vi "deadbands and cubic drive.vi"(8 "Axis2":dbl, 11 "Axis1":dbl) -> (0 "Axis2":dbl, 3 "Axis1":dbl)   [LabVIEW 2017]
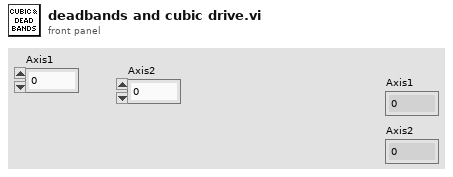
[diagram p1: front panel]
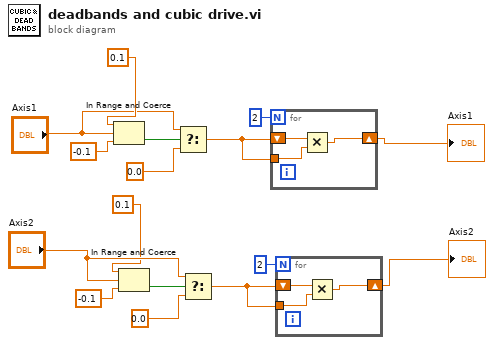
[diagram p0: block diagram]
diagram:
  n1 = In Range and Coerce(upper limit=0.1, x="Axis1", lower limit=-0.1) -> (In Range?=w14:bool)  [unwired: 1 out]
  n2 = In Range and Coerce(upper limit=0.1, x="Axis2", lower limit=-0.1) -> (In Range?=w5:bool)  [unwired: 1 out]
  n3 = Select(t="Axis1", s=w14, f=0.0) -> (s? t:f=w10:dbl)
  n4 = Select(t="Axis2", s=w5, f=0.0) -> (s? t:f=w8:dbl)
  n5 = for {
    N: 2 -> [_]
    tunnel: w10 -> [w18]
    shift-right: [w17] -> w9
    shift-left: w10 -> [w19]
    n6 = Multiply(x=w19, y=w18) -> (x*y=w17:dbl)
  }
  "Axis1" <- w9
  n7 = for {
    N: 2 -> [_]
    tunnel: w8 -> [w21]
    shift-right: [w20] -> w2
    shift-left: w8 -> [w22]
    n8 = Multiply(x=w22, y=w21) -> (x*y=w20:dbl)
  }
  "Axis2" <- w2
